vi "WaitString.vi"(2 "String to Receive":string, 3 "String to Send":string, 4 "PortNumber":i32=7) -> (0 "OK Done":bool, 1 "String Received":string)   [LabVIEW 2015]
panel:
  # "Port Number 0=COM1"
  # "Send the 'String to Send' to the Stage Controller and wait for the 'String to Receive'.\nAn Error occurs when received a different string or timed out."
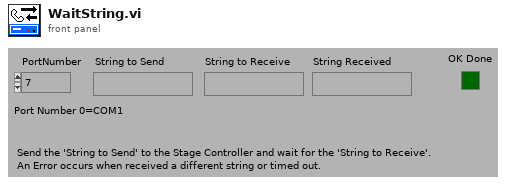
[diagram p1: front panel]
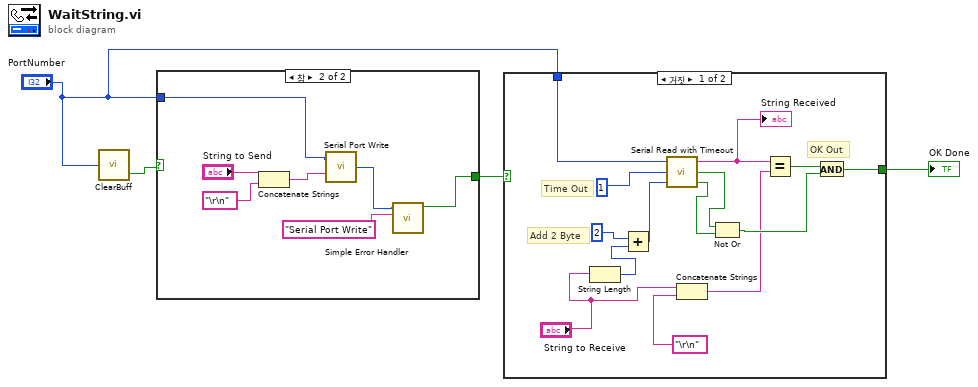
[diagram p0: block diagram]
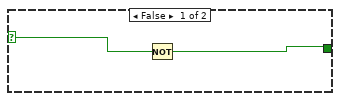
[diagram p2: hidden frame]
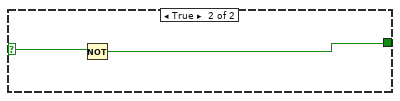
[diagram p3: hidden frame]
diagram:
  n1 = call "ClearBuff.vi"("PortNumber"="PortNumber") -> ("OK Done"=w2:bool)  [unwired: 1 out]
  n2 = case shown="참" w2 {
    selector: w2 -> [w6 _]
    tunnel: "PortNumber" -> [_ w7]
    tunnel: [w5 w8] -> w4
    frame False {
      n3 = Not(x=w6) -> (.not. x?=w5:bool)
    }
    frame True {
      n4 = Concatenate Strings("String to Send", "\r\n") -> (w11:string)
      n5 = call <vilib>:"Serial Port Write.vi"("string to write"=w11, "port number"=w7) -> ("error code"=w9:i32)
      n6 = call <vilib>:"Simple Error Handler.vi"("error code (no error:0)"=w9, "error source (\" \")"="Serial Port Write") -> ("error?"=w8:bool)  [unwired: 2 in, 5 out]
    }
  }
  n7 = case shown="거짓" w4 {
    selector: w4 -> [_ w29]
    tunnel: [w22 w28] -> w3
    tunnel: "PortNumber" -> [w14 _]
    frame False {
      # "OK Out"
      # "Time Out"
      # "Add 2 Byte"
      n8 = String Length(string="String to Receive") -> (length=w20:i32)
      n9 = Add(x=2, y=w20) -> (x+y=w18:i32)
      n10 = call "Serial Read with Timeout.vi"("Bytes to Read"=w18, "Timeout Limit"=1, "Port Number"=w14) -> ("Error Out"=w25:bool, "Timeout"=w26:bool, "Serial Read"=w21:string)
      "String Received" <- w21
      n11 = Concatenate Strings("String to Receive", "\r\n") -> (w15:string)
      n12 = Not Or(1:w25, 2:w26) -> (0:w23:bool)
      n13 = Equal?(x=w21, y=w15) -> (x = y?=w24:bool)
      n14 = And(x=w24, y=w23) -> (x .and. y?=w22:bool)
    }
    frame True {
      n15 = Not(x=w29) -> (.not. x?=w28:bool)
    }
  }
  "OK Done" <- w3
